vi "ProcessLoadSetData.vi"(8 "error in (no error)":errorcluster, 11 "MPC_VirbVision in":refnum<class "MPC_VirbVision.lvclass">) -> (0 "error out":errorcluster, 3 "MPC_VirbVision out":refnum<class "MPC_VirbVision.lvclass">)   [LabVIEW 2019, in "MPC_VirbVision.lvclass"]
uses:
  MPC_VirbVision.lvclass
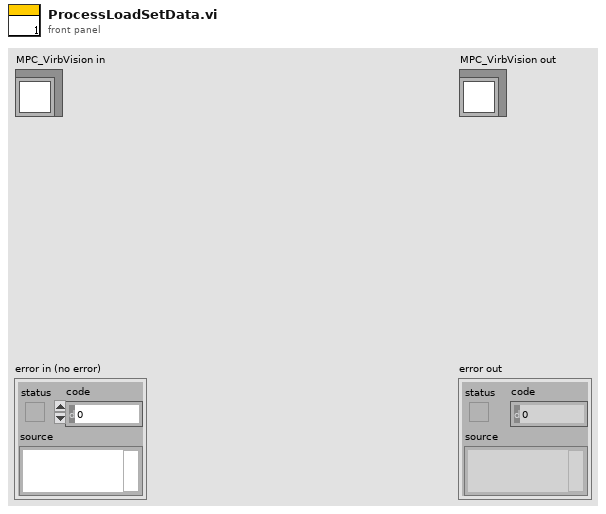
[diagram p1: front panel]
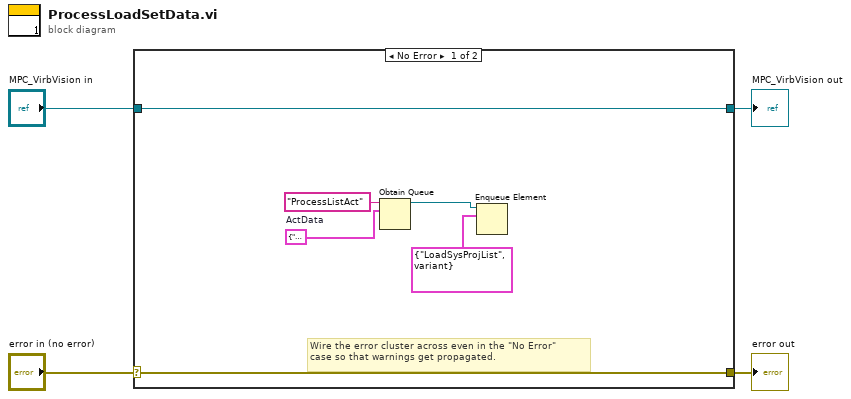
[diagram p0: block diagram]
diagram:
  n1 = case shown="No Error" "error in (no error)" {
    selector: "error in (no error)" -> [w9 w12]
    tunnel: [w9 w12] -> w3
    tunnel: [w10 w11] -> w1
    tunnel: "MPC_VirbVision in" -> [w10 w11]
    frame No Error {
      w5 = cluster{"Action":string, "Data":variant} {"Action"="", "Data"=variant}  # ActData
      # "Wire the error cluster across even in the \"No Error\"\ncase so that warnings get propagated."
      n2 = Obtain Queue(name (unnamed)="ProcessListAct", element data type=w5) -> (queue out=w8:refnum<queue>)  [unwired: 3 in, 2 out]
      n3 = Enqueue Element(queue=w8, element=cluster{"Action":string, "Data":variant} {"Action"="LoadSysProjList", "Data"=variant}) -> ()  [unwired: 2 in, 3 out]
    }
    frame Error {
    }
  }
  "error out" <- w3
  "MPC_VirbVision out" <- w1
